vi "ReadFlushBuffer.vi"(0 "object in":refnum<class "CoriFlowBFS1Plus.lvclass">, 5 "error in (no error)":errorcluster) -> (14 "object out":refnum<class "CoriFlowBFS1Plus.lvclass">, 16 "Buffer":T1(array[cluster]), 19 "error out":errorcluster)   [LabVIEW 2021, in "CoriFlowBFS1Plus.lvclass"]
uses:
  CoriFlowBFS1Plus.lvclass
  CoriFlowBFS1Plus.lvclass/CoriFlowBFS1Plus.ctl
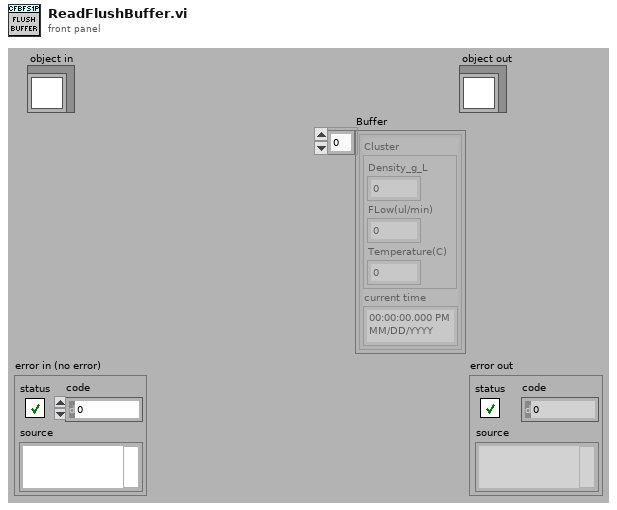
[diagram p1: front panel]
types:
  T1 = cluster{"Cluster":cluster{"Density_g_L":sgl, "FLow(ul/min)":sgl, "Temperature(C)":sgl}, "current time":timestamp}[]
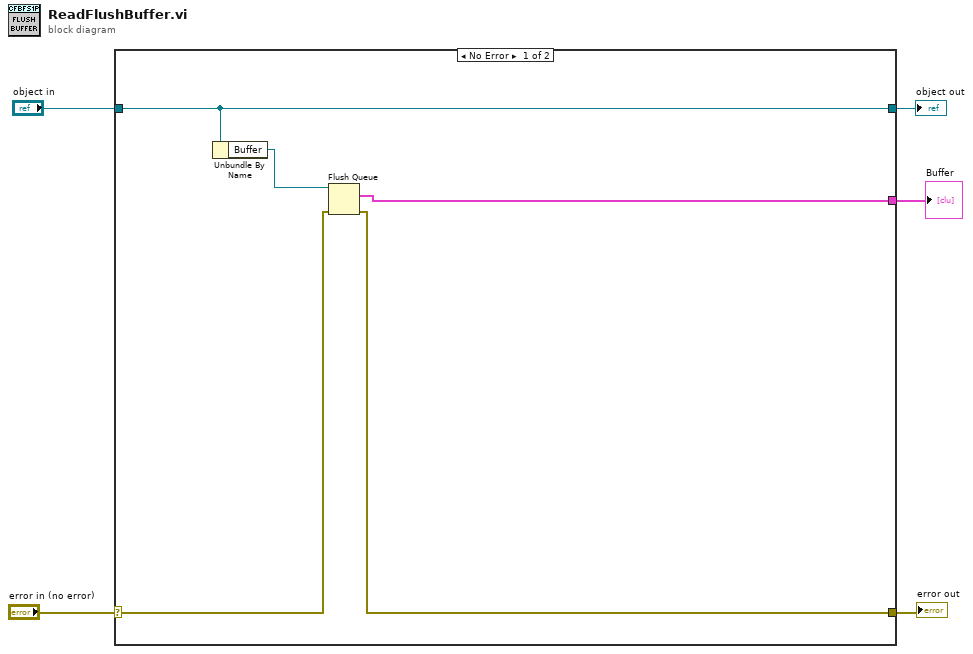
[diagram p0: block diagram]
diagram:
  n1 = case shown="No Error" "error in (no error)" {
    selector: "error in (no error)" -> [w8 w12]
    tunnel: [w7 w12] -> w4
    tunnel: [w10 w11] -> w2
    tunnel: "object in" -> [w10 w11]
    tunnel: [w6 _] -> w1
    frame No Error {
      n2 = Unbundle By Name(w10) -> ("Buffer"=w9:refnum<queue>)
      n3 = Flush Queue(queue=w9, error in (no error)=w8) -> (remaining elements=w6:T1, error out=w7:errorcluster)  [unwired: 1 out]
    }
    frame Error {
    }
  }
  "error out" <- w4
  "object out" <- w2
  "Buffer" <- w1
